vi "Agilent SNA Set Display Data.vi"(6 "Channel":i8=1 min=1 max=99 step=1, 7 "Agilent SNA & SWP":T3, 8 "error in (no error)":errorcluster, 10 "Display Data":T1, 11 "VISA Resource Names":T2) -> (0 "error out":errorcluster, 3 "dup VISA Resource Names":T2)   [LabVIEW 2011]
uses:
  TypeDefs/Agilent SNA Instrument Info.ctl
  TypeDefs/Agilent SNA VISA.ctl
  TypeDefs/Agilent SNA Display Data.ctl
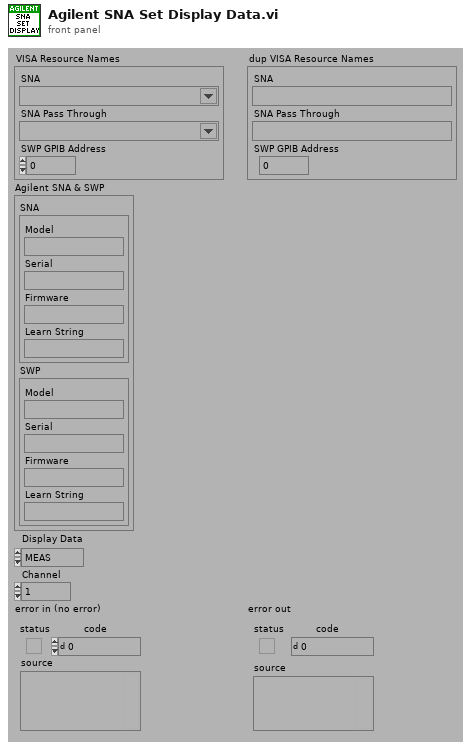
[diagram p1: front panel]
types:
  T1 = typedef "Agilent SNA Display Data.ctl" = enum16{"MEAS", "MEM", "MEAS-MEM"}
  T2 = typedef "Agilent SNA VISA.ctl" = cluster{"SNA":refnum<visa-resource-name>, "SNA Pass Through":refnum<visa-resource-name>, "SWP GPIB Address":i32}
  T3 = typedef "Agilent SNA Instrument Info.ctl" = cluster{"SNA":cluster{"Model":string, "Serial":string, "Firmware":string, "Learn String":string}, "SWP":cluster{"Model":string, "Serial":string, "Firmware":string, "Learn String":string}}
  T4 = typedef "Agilent SNA Model.ctl" = enum16{"Not Supported", "8757X"}
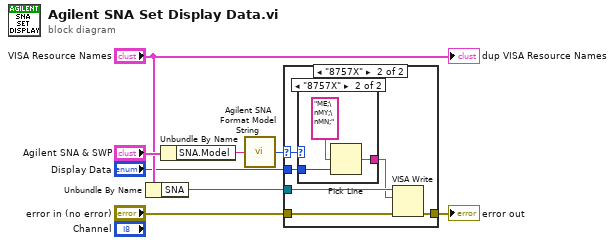
[diagram p0: block diagram]
diagram:
  n1 = Unbundle By Name("VISA Resource Names") -> ("SNA"=w2:refnum<visa-resource-name>)
  n2 = Unbundle By Name("Agilent SNA & SWP") -> ("SNA.Model"=w5:string)
  n3 = call "Agilent SNA Format Model String.vi"("Model String"=w5) -> ("Model"=w6:T4)
  n4 = case shown="\"8757X\"" w6 {
    selector: w6 -> [_ w14]
    tunnel: [w9 w15] -> w8
    tunnel: w2 -> [_ w13]
    tunnel: "error in (no error)" -> [w9 w12]
    tunnel: "Display Data" -> [_ w10]
    frame "Not Supported" {
    }
    frame "8757X" {
      n5 = case shown="\"8757X\"" w14 {
        tunnel: [_ w17] -> w11
        tunnel: w10 -> [_ w16]
        frame "Not Supported" {
        }
        frame "8757X" {
          n6 = Pick Line(multi-line string="ME;\nMY;\nMN;", line index=w16) -> (output string=w17:string)  [unwired: 1 out]
        }
      }
      n7 = VISA Write(VISA resource name=w13, write buffer=w11, error in (no error)=w12) -> (error out=w15:errorcluster)  [unwired: 2 out]
    }
  }
  "error out" <- w8
  "dup VISA Resource Names" <- "VISA Resource Names"
